vi "torreHanoi_v2.vi"() -> ()   [LabVIEW 2020]
uses:
  <vilib>/Analysis/Matrix/Datatypes/RealMatrix.ctl
  <vilib>/Utility/miscctls.llb/LVPositionTypeDef.ctl
  <vilib>/Utility/miscctls.llb/LVBoundsTypeDef.ctl
  <vilib>/Analysis/Matrix/NI_Matrix.lvlib
panel:
  out "PosAntPiezaCuatro":T1
  out "PosAntPiezaTres":T1
  out "PosAntPiezaDos":T1
  out "PosAntPiezaCinco":T1
  out "Posicion":i32
  out "Torre":i8
  out "posPiezaDos":i32[][](array[numeric])
  out "posPiezaTres":i32[][](array[numeric])
  out "posPiezaUno":i32[][](array[numeric])
  out "posPiezaCinco":i32[](array[numeric])
  out "posPiezaCuatro":i32[][](array[numeric])
  out "estadoTorreTres":i32[](array[numeric])
  out "estadoTorreUno":i32[](array[numeric])
  out "estadoTorreDos":i32[](array[numeric])
  out "PosAntPiezaUno":T1
  out "¿Pieza?":i8
  out "matrizPosIniciales":T2
  out "numMov":dbl
  out "minMov":dbl
  in  "numPiezas":enum16{"5", "4", "3"}(ring)
  in  "Iniciar":bool
  out "PiezaCinco":bool
  out "PiezaCuatro":bool
  out "PiezaTres":bool
  out "PiezaDos":bool
  in  "Deterner":bool
  out "PiezaUno":bool
  out "TorreUno":u8(slide) scale=0.0..100.0
  out "TorreDos":u8(slide) scale=0.0..100.0
  out "TorreTres":u8(slide) scale=0.0..100.0
  # "Número de Piezas"
  # "Minimo de Movimientos"
  # "Tus Movimientos"
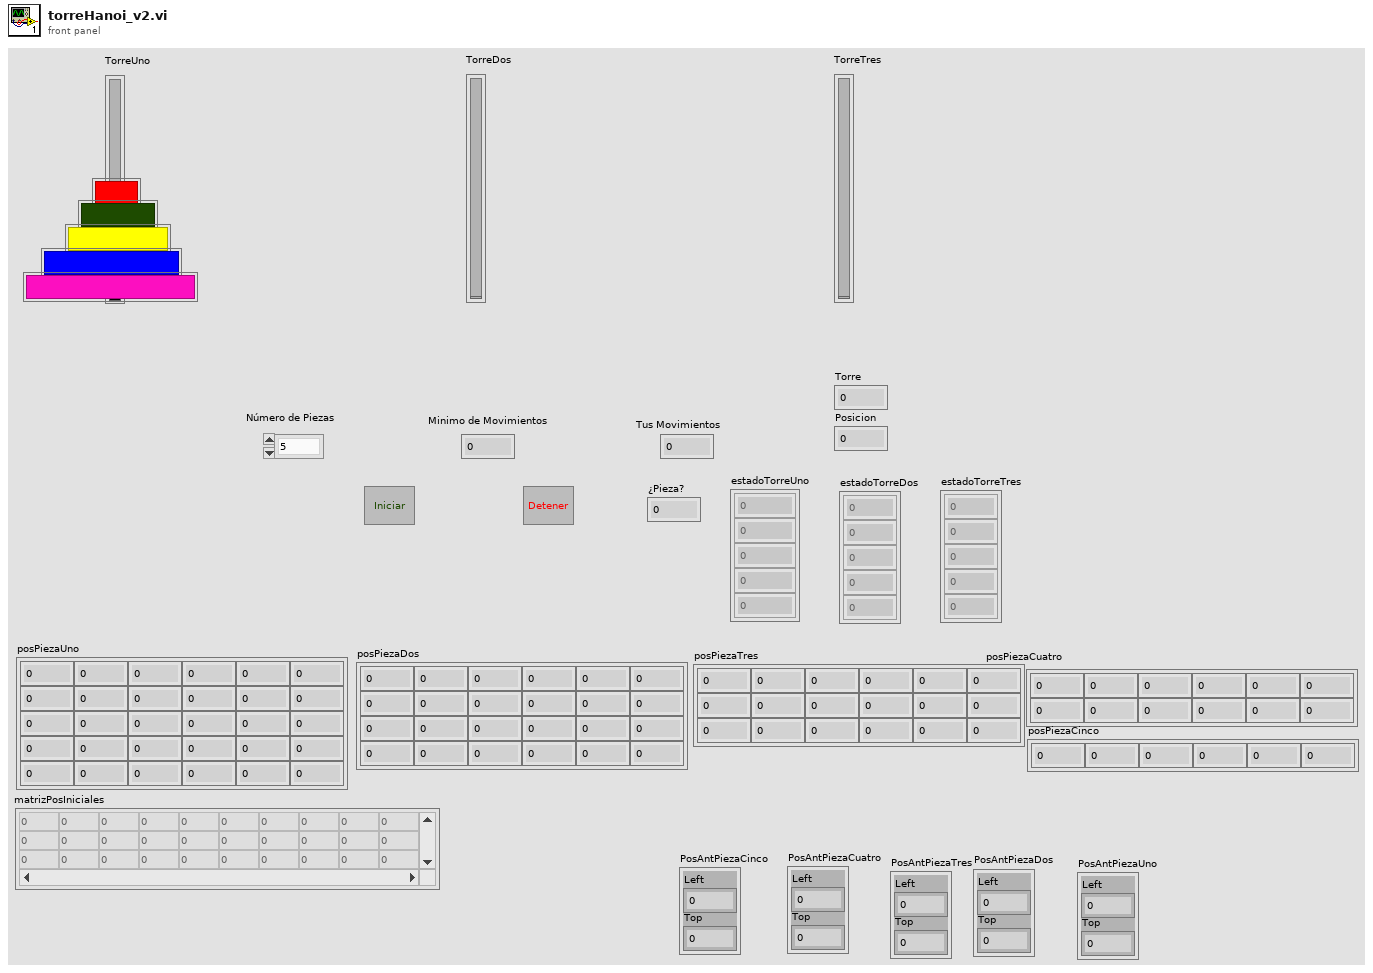
[diagram p1: front panel]
types:
  T1 = typedef "LVPositionTypeDef.ctl" = cluster{"Left":i32, "Top":i32}
  T2 = typedef "NI_Matrix.lvlib/RealMatrix.ctl" = dbl[][]
  T3 = typedef "LVBoundsTypeDef.ctl" = cluster{"Width":u32, "Height":u32}
  T4 = typedef "LVPoint32TypeDef.ctl" = cluster{"Horizontal":i32, "Vertical":i32}
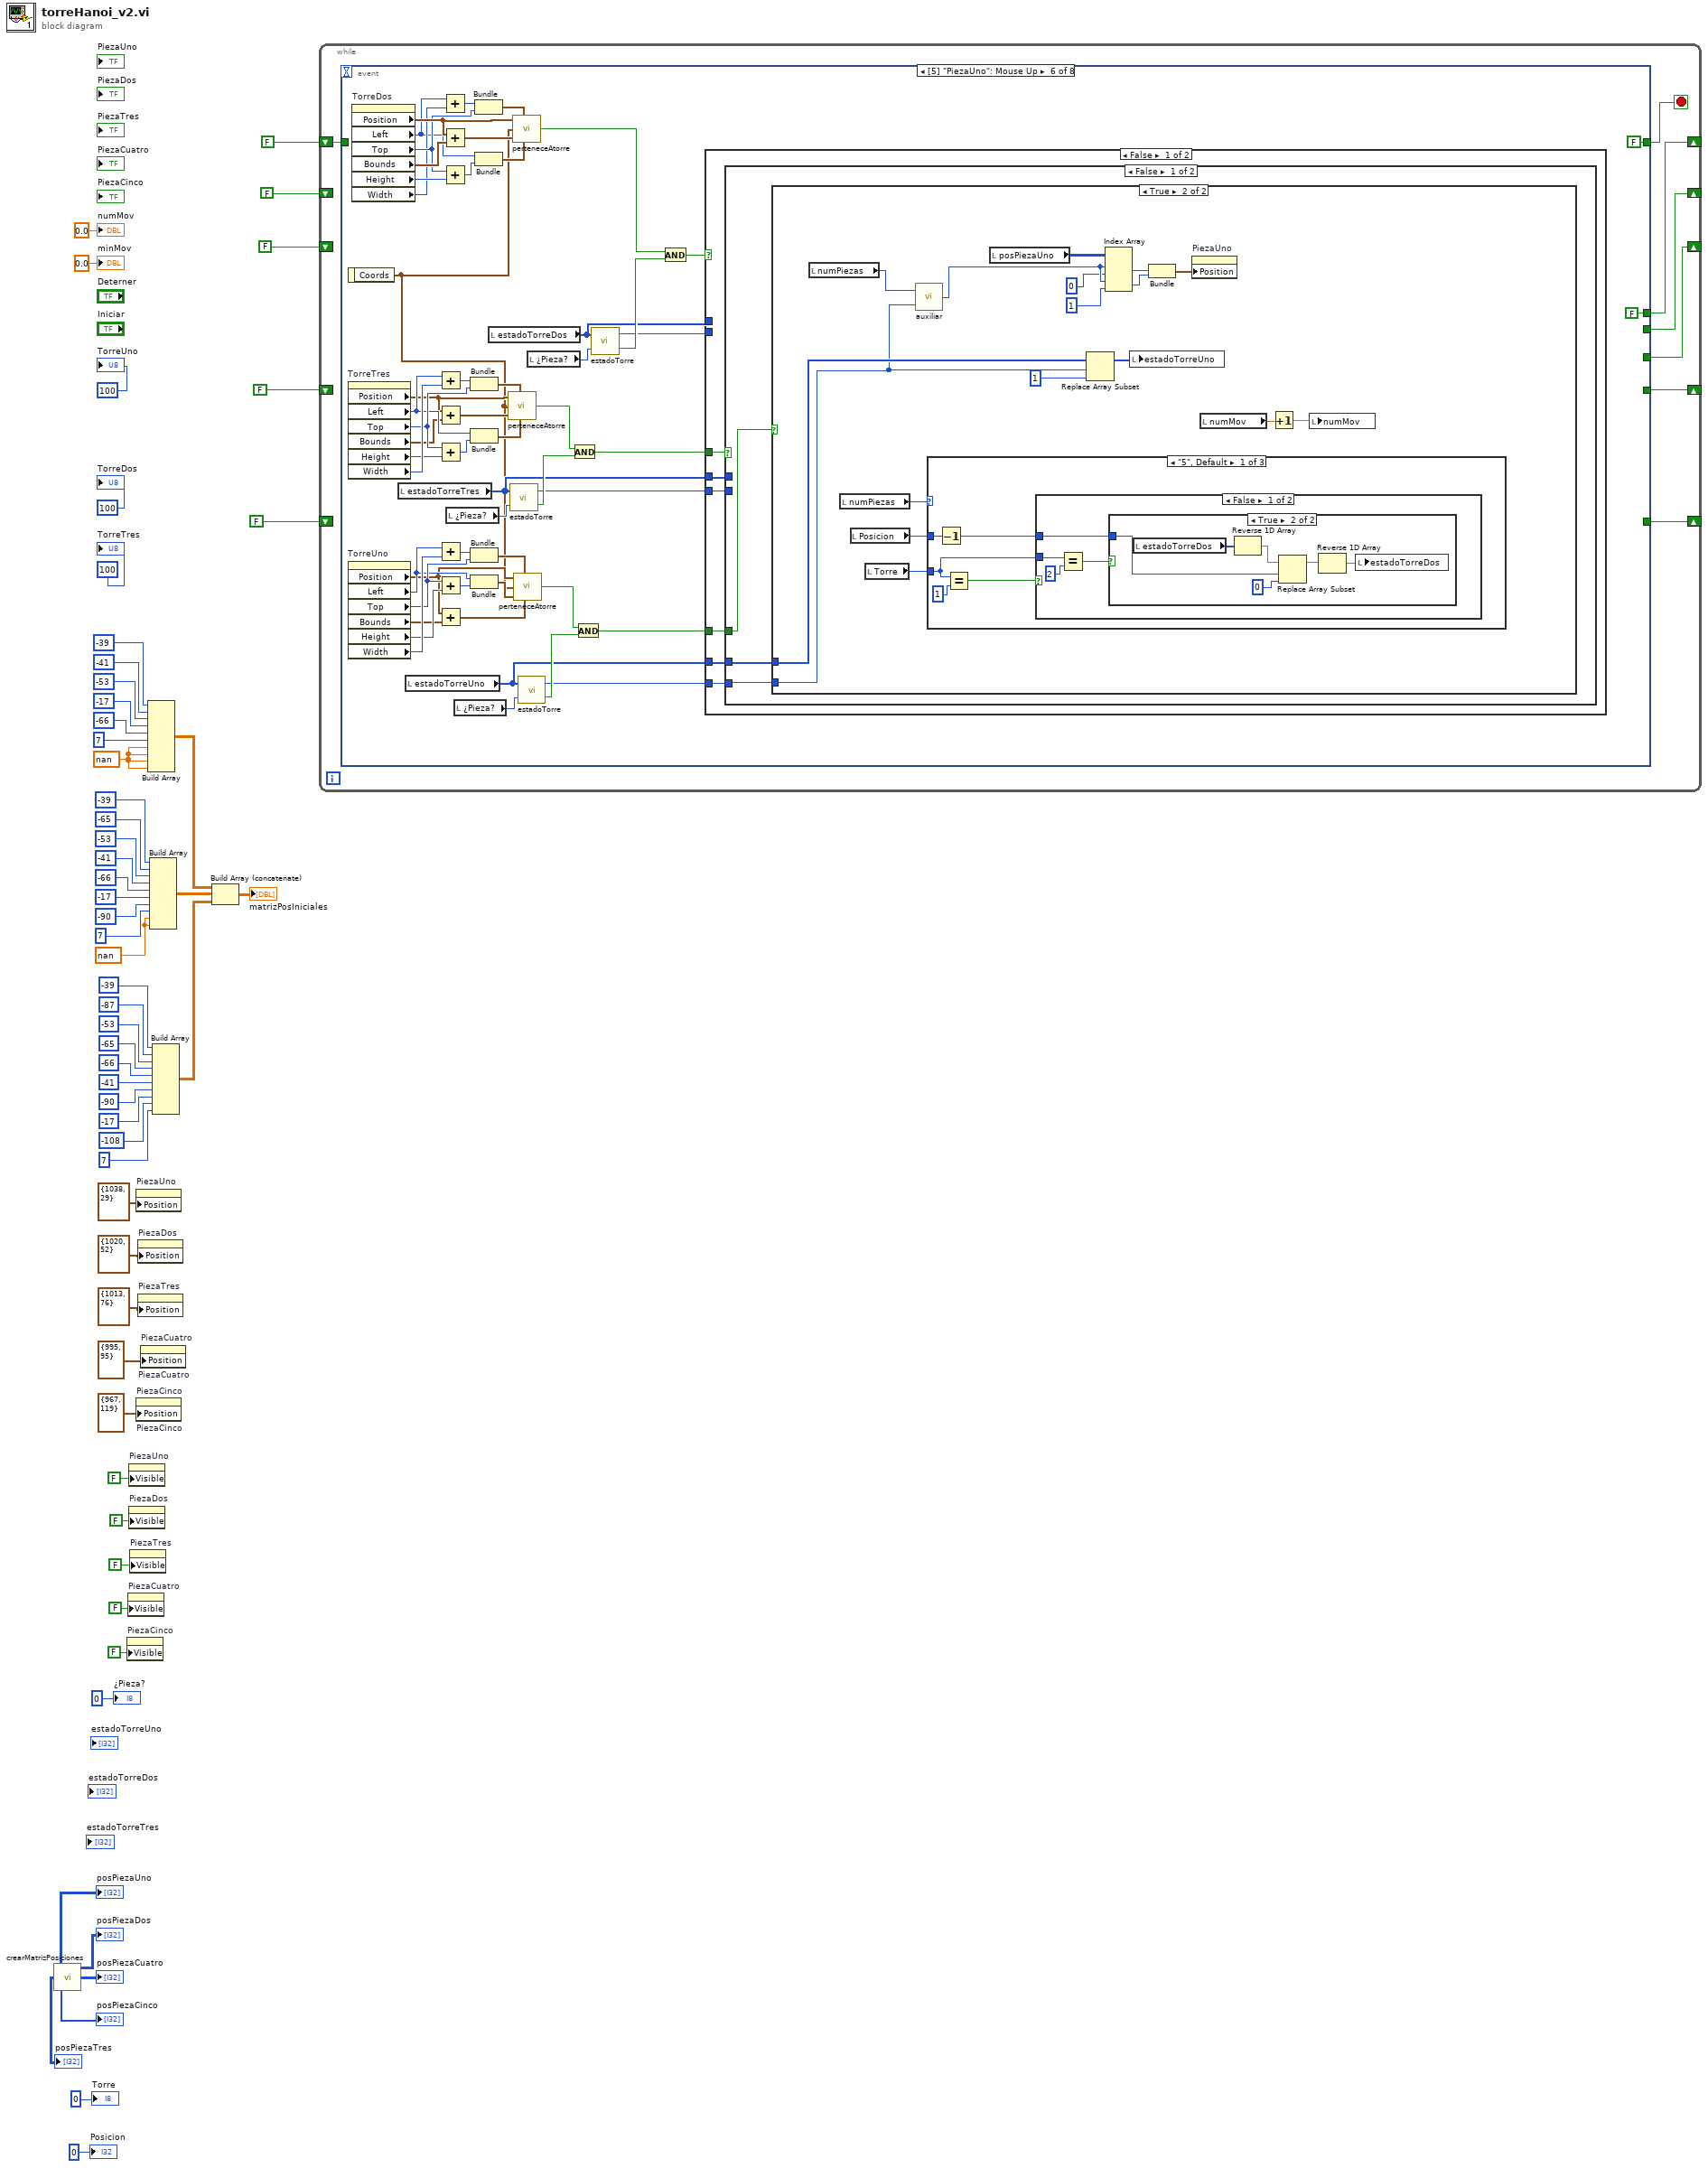
[diagram p0: block diagram]
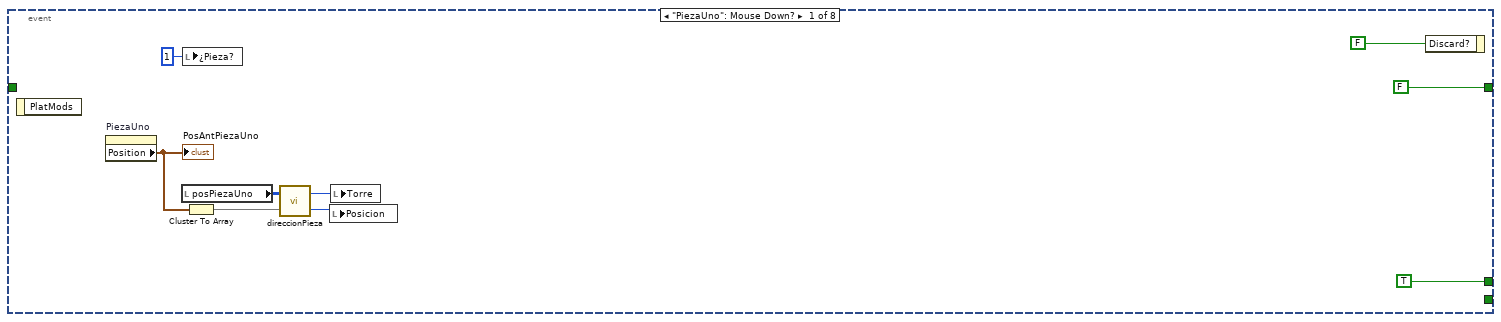
[diagram p2: hidden frame]
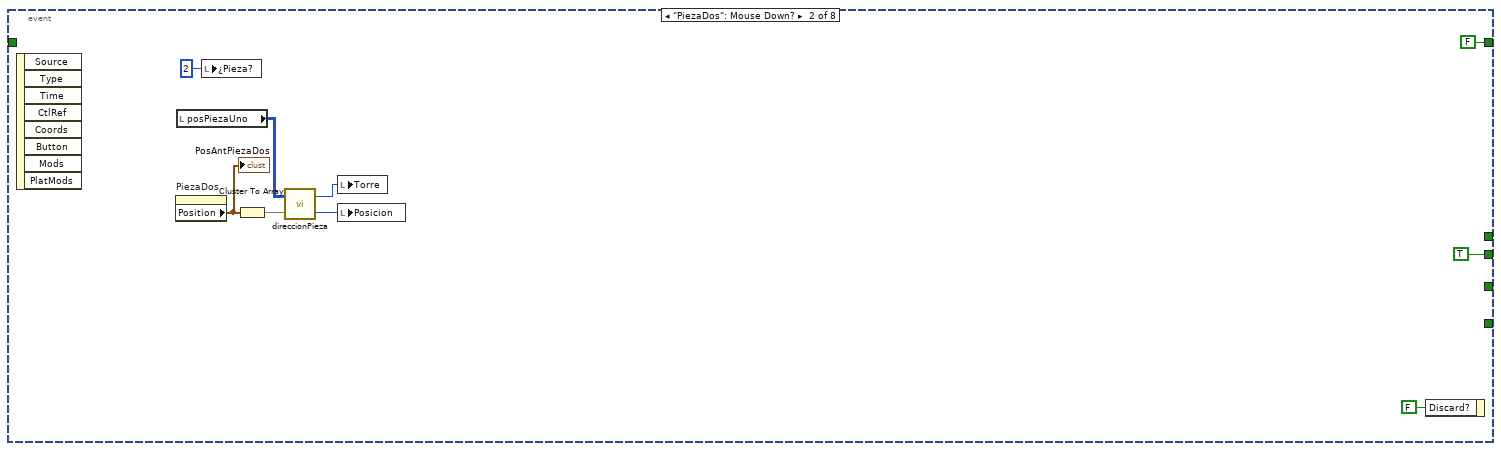
[diagram p3: hidden frame]
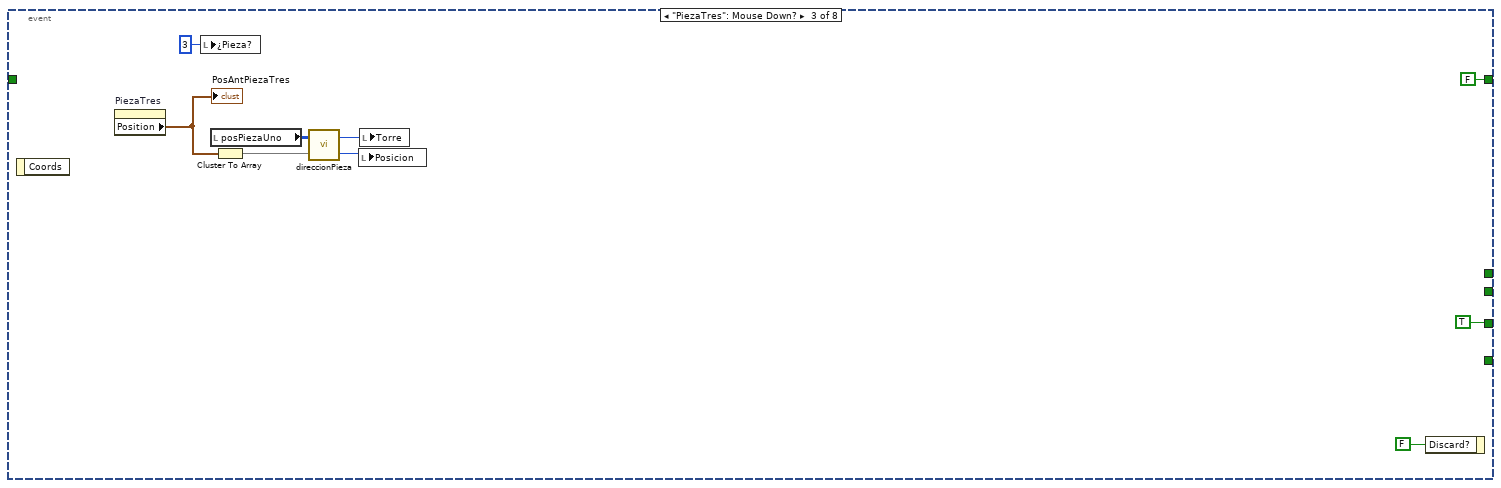
[diagram p4: hidden frame]
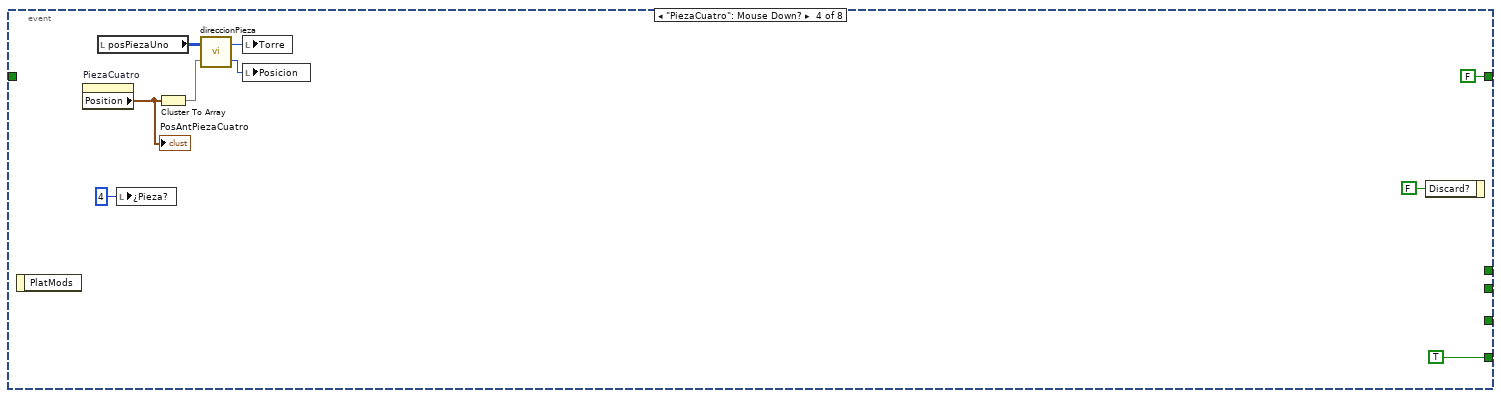
[diagram p5: hidden frame]
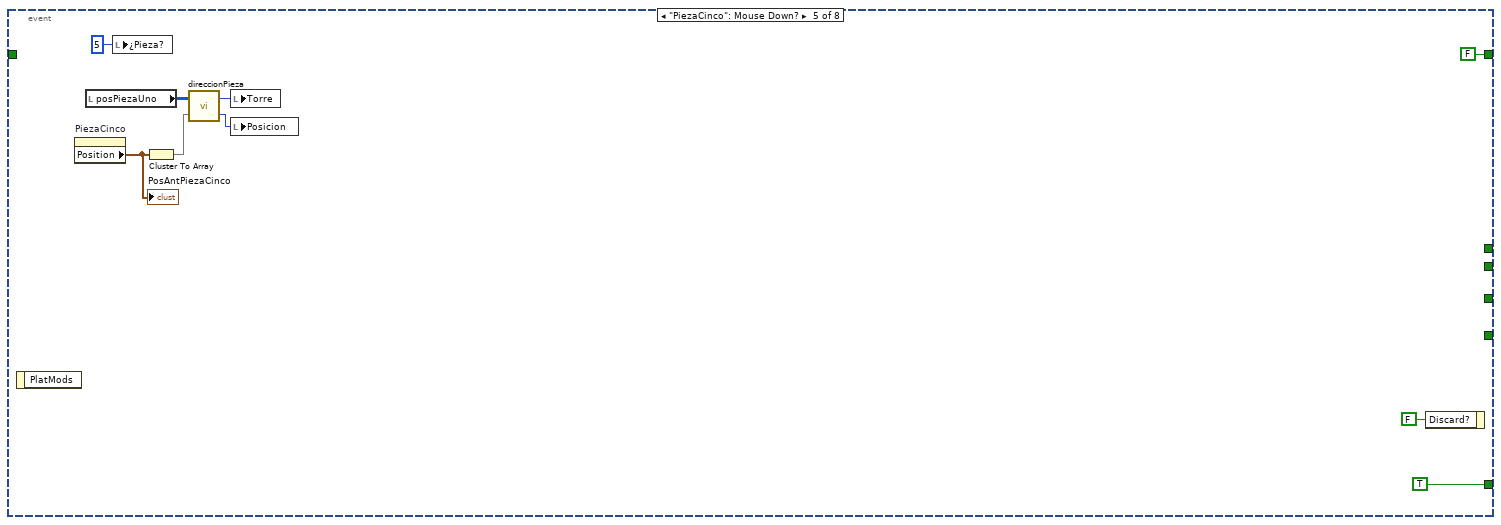
[diagram p6: hidden frame]
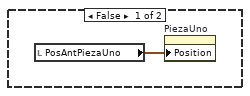
[diagram p7: hidden frame]
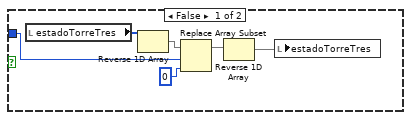
[diagram p8: hidden frame]
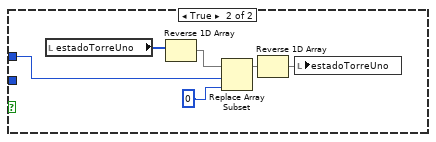
[diagram p9: hidden frame]
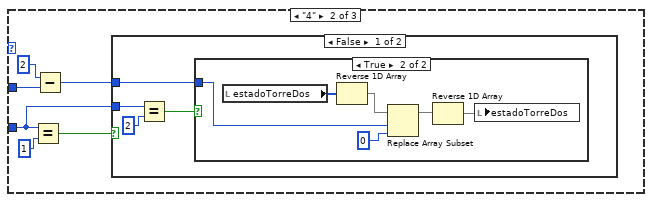
[diagram p10: hidden frame]
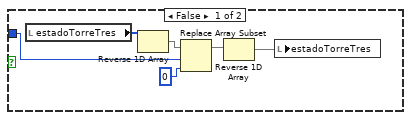
[diagram p11: hidden frame]
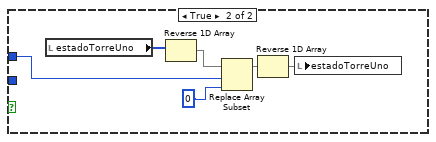
[diagram p12: hidden frame]
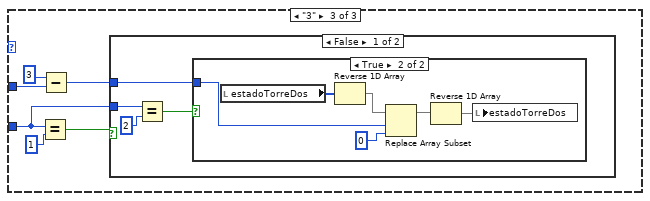
[diagram p13: hidden frame]
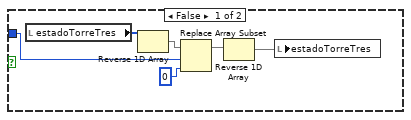
[diagram p14: hidden frame]
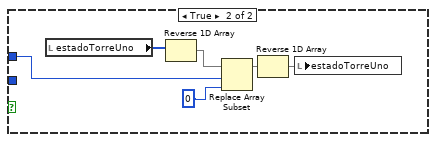
[diagram p15: hidden frame]
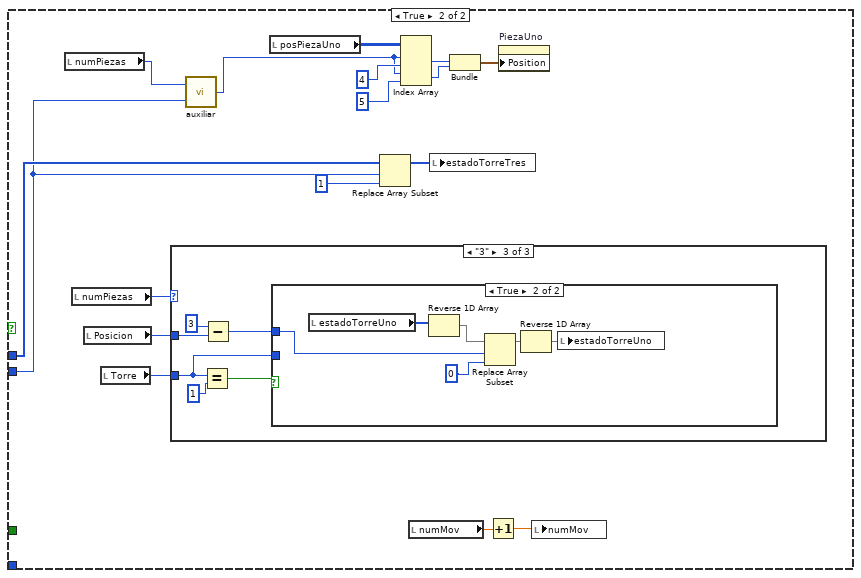
[diagram p16: hidden frame]
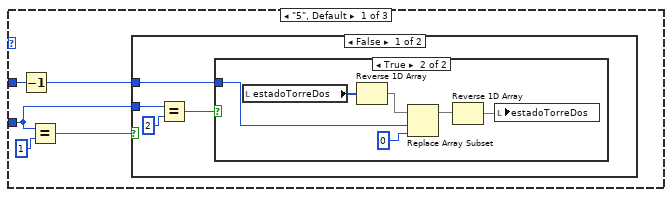
[diagram p17: hidden frame]
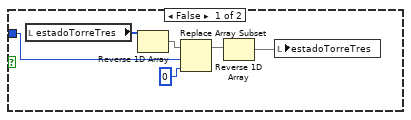
[diagram p18: hidden frame]
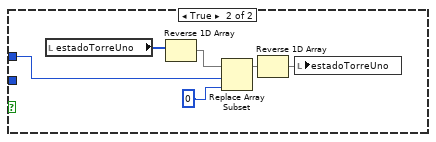
[diagram p19: hidden frame]
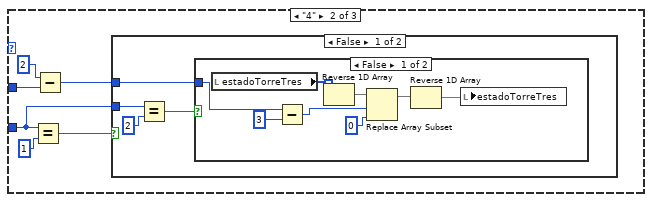
[diagram p20: hidden frame]
diagram:
  w41 = nan
  w50 = nan
  n1 = call "crearMatrizPosiciones.vi"() -> ("posPiezaCuatro"=→"posPiezaCuatro":i32[][], "posPiezaDos"=→"posPiezaDos":i32[][], "posPiezaCinco"=→"posPiezaCinco":i32[], "posPiezaTres"=→"posPiezaTres":i32[][], "posPiezaUno"=→"posPiezaUno":i32[][])  [unwired: 1 in]
  n2 = property on="PiezaCinco" class="Bool (strict)"("Visible"=FALSE ("PiezaCinco")) -> ()  [unwired: 2 in, 2 out]
  n3 = property on="PiezaCuatro" class="Bool (strict)"("Visible"=FALSE ("PiezaCuatro")) -> ()  [unwired: 2 in, 2 out]
  n4 = property on="PiezaUno" class="Bool (strict)"("Visible"=FALSE) -> ()  [unwired: 2 in, 2 out]
  n5 = property on="PiezaDos" class="Bool (strict)"("Visible"=FALSE ("PiezaDos")) -> ()  [unwired: 2 in, 2 out]
  n6 = property on="PiezaTres" class="Bool (strict)"("Visible"=FALSE) -> ()  [unwired: 2 in, 2 out]
  n7 = property on="PiezaUno" class="Bool (strict)"("Position"=T1 {"Left"=1038, "Top"=29}) -> ()  [unwired: 2 in, 2 out]
  n8 = property on="PiezaCinco" class="Bool (strict)"("Position"=T1 {"Left"=967, "Top"=119}) -> ()  [unwired: 2 in, 2 out]
  n9 = property on="PiezaCinco" class="Bool (strict)"("Position"=T1 {"Left"=967, "Top"=119}) -> ()  [unwired: 2 in, 2 out]
  n10 = property on="PiezaDos" class="Bool (strict)"("Position"=T1 {"Left"=1020, "Top"=52}) -> ()  [unwired: 2 in, 2 out]
  n11 = property on="PiezaTres" class="Bool (strict)"("Position"=T1 {"Left"=1013, "Top"=76}) -> ()  [unwired: 2 in, 2 out]
  n12 = property on="PiezaCuatro" class="Bool (strict)"("Position"=T1 {"Left"=995, "Top"=95}) -> ()  [unwired: 2 in, 2 out]
  n13 = property on="PiezaCuatro" class="Bool (strict)"("Position"=T1 {"Left"=995, "Top"=95}) -> ()  [unwired: 2 in, 2 out]
  n14 = Build Array(-39, -41 ("element"), -53 ("element"), -17 ("element"), -66 ("element"), 7 ("element"), w50, w50, w50, w50) -> (w30:T2)
  n15 = Build Array(-39, -65 ("element"), -53 ("element"), -41 ("element"), -66 ("element"), -17 ("element"), -90 ("element"), 7 ("element"), w41, w41) -> (w29:T2)
  n16 = Build Array(-39, -87 ("element"), -53 ("element"), -65 ("element"), -66 ("element"), -41 ("element"), -90 ("element"), -17 ("element"), -108 ("element"), 7 ("element")) -> (w28:T2)
  n17 = Build Array (concatenate)(w30, w29, w28) -> (→"matrizPosIniciales":T2)
  n18 = while {
    shift-right: [w66] -> _
    shift-left: FALSE -> [w65]
    shift-right: [w64] -> _
    shift-left: FALSE -> [_]
    shift-right: [w63] -> _
    shift-left: FALSE -> [_]
    shift-right: [w62] -> _
    shift-left: FALSE -> [_]
    shift-right: [w61] -> _
    shift-left: FALSE -> [_]
    stop <- w67 stop-if-true
    n19 = event shown="[5] \"PiezaUno\": Mouse Up" {
      selector: _ -> [_ _ _ _ _ _ _ _]
      dyn-events: _ -> [_ _ _ _ _ _ _ _]
      timeout: _ -> [_ _ _ _ _ _ _ _]
      tunnel: [FALSE FALSE FALSE FALSE FALSE FALSE FALSE _] -> w67
      tunnel: [TRUE _ _ _ _ FALSE w480 _] -> w66
      tunnel: w65 -> [_ _ _ _ _ _ w480 _]
      tunnel: [_ TRUE _ _ _ _ _ _] -> w64
      tunnel: [_ _ TRUE _ _ _ _ _] -> w63
      tunnel: [_ _ _ TRUE _ _ _ _] -> w62
      tunnel: [_ _ _ _ TRUE _ _ _] -> w61
      event "PiezaUno": Mouse Down? {
        n20 = event-data() -> ()  [unwired: 1 in, 1 out]
        n21 = property on="PiezaUno" class="Bool (strict)"() -> ("Position"=w72:T1)  [unwired: 2 in, 2 out]
        "PosAntPiezaUno" <- w72
        n22 = local read "posPiezaUno"() -> (w70:i32[][])
        n23 = local write "¿Pieza?"(i8 1 ("¿Pieza?")) -> ()
        n24 = Cluster To Array(cluster=w72) -> (array=w71:i32[])
        n25 = call "direccionPieza.vi"("posicion"=w71, "matrizPosiciones"=w70) -> ("Posicion"=w69:i32, "Torre"=w68:i8)
        n26 = local write "Posicion"(w69) -> ()
        n27 = local write "Torre"(w68) -> ()
        n28 = event-data("Discard?"=FALSE) -> ()  [unwired: 1 in, 1 out]
      }
      event "PiezaDos": Mouse Down? {
        n29 = event-data() -> ()  [unwired: 1 in, 8 out]
        n30 = property on="PiezaDos" class="Bool (strict)"() -> ("Position"=w80:T1)  [unwired: 2 in, 2 out]
        "PosAntPiezaDos" <- w80
        n31 = local read "posPiezaUno"() -> (w82:i32[][])
        n32 = local write "¿Pieza?"(i8 2 ("¿Pieza?")) -> ()
        n33 = Cluster To Array(cluster=w80) -> (array=w81:i32[])
        n34 = call "direccionPieza.vi"("posicion"=w81, "matrizPosiciones"=w82) -> ("Posicion"=w83:i32, "Torre"=w84:i8)
        n35 = local write "Torre"(w84) -> ()
        n36 = local write "Posicion"(w83) -> ()
        n37 = event-data("Discard?"=FALSE) -> ()  [unwired: 1 in, 1 out]
      }
      event "PiezaTres": Mouse Down? {
        n38 = event-data() -> ()  [unwired: 1 in, 1 out]
        n39 = property on="PiezaTres" class="Bool (strict)"() -> ("Position"=w89:T1)  [unwired: 2 in, 2 out]
        "PosAntPiezaTres" <- w89
        n40 = local write "¿Pieza?"(i8 3 ("¿Pieza?")) -> ()
        n41 = local read "posPiezaUno"() -> (w91:i32[][])
        n42 = Cluster To Array(cluster=w89) -> (array=w90:i32[])
        n43 = call "direccionPieza.vi"("posicion"=w90, "matrizPosiciones"=w91) -> ("Posicion"=w92:i32, "Torre"=w93:i8)
        n44 = local write "Posicion"(w92) -> ()
        n45 = local write "Torre"(w93) -> ()
        n46 = event-data("Discard?"=FALSE) -> ()  [unwired: 1 in, 1 out]
      }
      event "PiezaCuatro": Mouse Down? {
        n47 = event-data() -> ()  [unwired: 1 in, 1 out]
        n48 = property on="PiezaCuatro" class="Bool (strict)"() -> ("Position"=w99:T1)  [unwired: 2 in, 2 out]
        "PosAntPiezaCuatro" <- w99
        n49 = local read "posPiezaUno"() -> (w101:i32[][])
        n50 = local write "¿Pieza?"(i8 4 ("¿Pieza?")) -> ()
        n51 = Cluster To Array(cluster=w99) -> (array=w100:i32[])
        n52 = call "direccionPieza.vi"("posicion"=w100, "matrizPosiciones"=w101) -> ("Posicion"=w102:i32, "Torre"=w103:i8)
        n53 = local write "Torre"(w103) -> ()
        n54 = local write "Posicion"(w102) -> ()
        n55 = event-data("Discard?"=FALSE) -> ()  [unwired: 1 in, 1 out]
      }
      event "PiezaCinco": Mouse Down? {
        n56 = event-data() -> ()  [unwired: 1 in, 1 out]
        n57 = property on="PiezaCinco" class="Bool (strict)"() -> ("Position"=w107:T1)  [unwired: 2 in, 2 out]
        "PosAntPiezaCinco" <- w107
        n58 = local read "posPiezaUno"() -> (w110:i32[][])
        n59 = local write "¿Pieza?"(i8 5 ("¿Pieza?")) -> ()
        n60 = Cluster To Array(cluster=w107) -> (array=w109:i32[])
        n61 = call "direccionPieza.vi"("posicion"=w109, "matrizPosiciones"=w110) -> ("Posicion"=w111:i32, "Torre"=w112:i8)
        n62 = local write "Torre"(w112) -> ()
        n63 = local write "Posicion"(w111) -> ()
        n64 = event-data("Discard?"=FALSE) -> ()  [unwired: 1 in, 1 out]
      }
      event "PiezaUno": Mouse Up {
        n65 = event-data() -> ("Coords"=w119:T4)  [unwired: 1 in]
        n66 = property on="TorreTres" class="Slide (strict)"() -> ("Position"=w138:T1, "Left"=w141:i32, "Top"=w144:i32, "Bounds"=w139:T3, "Height"=w143:u32, "Width"=w147:u32)  [unwired: 2 in, 2 out]
        n67 = property on="TorreUno" class="Slide (strict)"() -> ("Position"=w122:T1, "Left"=w124:i32, "Top"=w127:i32, "Bounds"=w121:T3, "Height"=w126:u32, "Width"=w130:u32)  [unwired: 2 in, 2 out]
        n68 = property on="TorreDos" class="Slide (strict)"() -> ("Position"=w161:T1, "Left"=w156:i32, "Top"=w159:i32, "Bounds"=w162:T3, "Height"=w158:u32, "Width"=w157:u32)  [unwired: 2 in, 2 out]
        n69 = local read "estadoTorreTres"() -> (w132:i32[])
        n70 = local read "estadoTorreUno"() -> (w113:i32[])
        n71 = Add(x=w141, y=w147) -> (x+y=w146:u32)
        n72 = Add(x=w138, y=w139) -> (x+y=w137:T3)
        n73 = Add(x=w144, y=w143) -> (x+y=w142:u32)
        n74 = Add(x=w124, y=w130) -> (x+y=w128:u32)
        n75 = Add(x=w127, y=w126) -> (x+y=w125:u32)
        n76 = Add(x=w122, y=w121) -> (x+y=w120:T3)
        n77 = Add(x=w156, y=w157) -> (x+y=w164:u32)
        n78 = Add(x=w161, y=w162) -> (x+y=w160:T3)
        n79 = Add(x=w159, y=w158) -> (x+y=w155:u32)
        n80 = local read "¿Pieza?"() -> (w136:i8)
        n81 = local read "¿Pieza?"() -> (w118:i8)
        n82 = Bundle(w146, "Top"=w144) -> (w145:cluster{u32, "Top":i32})  [unwired: 1 in]
        n83 = Bundle("Left"=w141, w142) -> (w140:cluster{"Left":i32, u32})  [unwired: 1 in]
        n84 = Bundle(w128, "Top"=w127) -> (w129:cluster{u32, "Top":i32})  [unwired: 1 in]
        n85 = Bundle("Left"=w124, w125) -> (w123:cluster{"Left":i32, u32})  [unwired: 1 in]
        n86 = Bundle(w164, "Top"=w159) -> (w163:cluster{u32, "Top":i32})  [unwired: 1 in]
        n87 = Bundle("Left"=w156, w155) -> (w154:cluster{"Left":i32, u32})  [unwired: 1 in]
        n88 = local read "estadoTorreDos"() -> (w148:i32[])
        n89 = call "perteneceAtorre.vi"("P1"=w138, "P2"=w145, "P"=w119, "P3"=w137, "P4"=w140) -> ("out"=w135:bool)
        n90 = call "estadoTorre.vi"("¿pieza?"=w136, "estadoTorre"=w132) -> ("¿disponible?"=w134:bool, "posicionCero"=w133:i32)
        n91 = call "perteneceAtorre.vi"("P1"=w161, "P2"=w163, "P"=w119, "P3"=w160, "P4"=w154) -> ("out"=w152:bool)
        n92 = call "perteneceAtorre.vi"("P1"=w122, "P2"=w129, "P"=w119, "P3"=w123, "P4"=w120) -> ("out"=w117:bool)
        n93 = call "estadoTorre.vi"("¿pieza?"=w118, "estadoTorre"=w113) -> ("¿disponible?"=w116:bool, "posicionCero"=w114:i32)
        n94 = local read "¿Pieza?"() -> (w151:i8)
        n95 = And(x=w135, y=w134) -> (x .and. y?=w131:bool)
        n96 = And(x=w117, y=w116) -> (x .and. y?=w115:bool)
        n97 = call "estadoTorre.vi"("¿pieza?"=w151, "estadoTorre"=w148) -> ("¿disponible?"=w150:bool, "posicionCero"=w149:i32)
        n98 = And(x=w152, y=w150) -> (x .and. y?=w153:bool)
        n99 = case shown="False" w153 {
          tunnel: w149 -> [_ w385]
          tunnel: w148 -> [_ w389]
          tunnel: w133 -> [w170 _]
          tunnel: w132 -> [w171 _]
          tunnel: w131 -> [w172 _]
          tunnel: w115 -> [w169 _]
          tunnel: w114 -> [w167 _]
          tunnel: w113 -> [w168 _]
          frame False {
            n100 = case shown="False" w172 {
              tunnel: w171 -> [_ w283]
              tunnel: w170 -> [_ w282]
              tunnel: w169 -> [w175 _]
              tunnel: w168 -> [w174 _]
              tunnel: w167 -> [w173 _]
              frame False {
                n101 = case shown="True" w175 {
                  tunnel: w174 -> [_ w183]
                  tunnel: w173 -> [_ w182]
                  frame False {
                    n102 = local read "PosAntPiezaUno"() -> (w176:T1)
                    n103 = property on="PiezaUno" class="Bool (strict)"("Position"=w176) -> ()  [unwired: 2 in, 2 out]
                  }
                  frame True {
                    n104 = local read "numPiezas"() -> (w188:enum16{"5", "4", "3"})
                    n105 = local read "numPiezas"() -> (w181:enum16{"5", "4", "3"})
                    n106 = local read "Posicion"() -> (w180:i32)
                    n107 = local read "Torre"() -> (w179:i8)
                    n108 = call "auxiliar.vi"("posicion"=w182, "numPiezas"=w188) -> ("posicion"=w187:i32)
                    n109 = case shown="\"5\", Default" w181 {
                      tunnel: w180 -> [w198 w224 w252]
                      tunnel: w179 -> [w195 w221 w249]
                      frame "5", Default {
                        n110 = Decrement(x=w198) -> (x-1=w194:i32)
                        n111 = Equal?(x=w195, y=i8 1) -> (x = y?=w196:bool)
                        n112 = case shown="False" w196 {
                          tunnel: w194 -> [w199 w219]
                          tunnel: w195 -> [w202 _]
                          frame False {
                            n113 = Equal?(x=w202, y=i8 2) -> (x = y?=w200:bool)
                            n114 = case shown="True" w200 {
                              tunnel: w199 -> [w207 w213]
                              frame False {
                                n115 = local read "estadoTorreTres"() -> (w204:i32[])
                                n116 = Reverse 1D Array(array=w204) -> (reversed array=w203:i32[])
                                n117 = Replace Array Subset(array=w203, new element=0 ("new element/subarray"), index=w207) -> (w206:i32[])
                                n118 = Reverse 1D Array(array=w206) -> (reversed array=w205:i32[])
                                n119 = local write "estadoTorreTres"(w205) -> ()
                              }
                              frame True {
                                n120 = local read "estadoTorreDos"() -> (w210:i32[])
                                n121 = Reverse 1D Array(array=w210) -> (reversed array=w209:i32[])
                                n122 = Replace Array Subset(array=w209, new element=0 ("new element/subarray"), index=w213) -> (w212:i32[])
                                n123 = Reverse 1D Array(array=w212) -> (reversed array=w211:i32[])
                                n124 = local write "estadoTorreDos"(w211) -> ()
                              }
                            }
                          }
                          frame True {
                            n125 = local read "estadoTorreUno"() -> (w216:i32[])
                            n126 = Reverse 1D Array(array=w216) -> (reversed array=w215:i32[])
                            n127 = Replace Array Subset(array=w215, new element=0 ("new element/subarray"), index=w219) -> (w218:i32[])
                            n128 = Reverse 1D Array(array=w218) -> (reversed array=w217:i32[])
                            n129 = local write "estadoTorreUno"(w217) -> ()
                          }
                        }
                      }
                      frame "4" {
                        n130 = Equal?(x=w221, y=i8 1) -> (x = y?=w226:bool)
                        n131 = Subtract(x=2, y=w224) -> (x-y=w223:i32)
                        n132 = case shown="False" w226 {
                          tunnel: w223 -> [w228 w247]
                          tunnel: w221 -> [w227 _]
                          frame False {
                            n133 = Equal?(x=w227, y=i8 2) -> (x = y?=w229:bool)
                            n134 = case shown="True" w229 {
                              tunnel: w228 -> [w235 w241]
                              frame False {
                                n135 = local read "estadoTorreTres"() -> (w232:i32[])
                                n136 = Reverse 1D Array(array=w232) -> (reversed array=w231:i32[])
                                n137 = Replace Array Subset(array=w231, new element=0 ("new element/subarray"), index=w235) -> (w234:i32[])
                                n138 = Reverse 1D Array(array=w234) -> (reversed array=w233:i32[])
                                n139 = local write "estadoTorreTres"(w233) -> ()
                              }
                              frame True {
                                n140 = local read "estadoTorreDos"() -> (w238:i32[])
                                n141 = Reverse 1D Array(array=w238) -> (reversed array=w237:i32[])
                                n142 = Replace Array Subset(array=w237, new element=0 ("new element/subarray"), index=w241) -> (w240:i32[])
                                n143 = Reverse 1D Array(array=w240) -> (reversed array=w239:i32[])
                                n144 = local write "estadoTorreDos"(w239) -> ()
                              }
                            }
                          }
                          frame True {
                            n145 = local read "estadoTorreUno"() -> (w244:i32[])
                            n146 = Reverse 1D Array(array=w244) -> (reversed array=w243:i32[])
                            n147 = Replace Array Subset(array=w243, new element=0 ("new element/subarray"), index=w247) -> (w246:i32[])
                            n148 = Reverse 1D Array(array=w246) -> (reversed array=w245:i32[])
                            n149 = local write "estadoTorreUno"(w245) -> ()
                          }
                        }
                      }
                      frame "3" {
                        n150 = Equal?(x=w249, y=i8 1) -> (x = y?=w254:bool)
                        n151 = Subtract(x=3, y=w252) -> (x-y=w250:i32)
                        n152 = case shown="False" w254 {
                          tunnel: w250 -> [w256 w275]
                          tunnel: w249 -> [w255 _]
                          frame False {
                            n153 = Equal?(x=w255, y=i8 2) -> (x = y?=w257:bool)
                            n154 = case shown="True" w257 {
                              tunnel: w256 -> [w263 w269]
                              frame False {
                                n155 = local read "estadoTorreTres"() -> (w260:i32[])
                                n156 = Reverse 1D Array(array=w260) -> (reversed array=w259:i32[])
                                n157 = Replace Array Subset(array=w259, new element=0 ("new element/subarray"), index=w263) -> (w262:i32[])
                                n158 = Reverse 1D Array(array=w262) -> (reversed array=w261:i32[])
                                n159 = local write "estadoTorreTres"(w261) -> ()
                              }
                              frame True {
                                n160 = local read "estadoTorreDos"() -> (w266:i32[])
                                n161 = Reverse 1D Array(array=w266) -> (reversed array=w265:i32[])
                                n162 = Replace Array Subset(array=w265, new element=0 ("new element/subarray"), index=w269) -> (w268:i32[])
                                n163 = Reverse 1D Array(array=w268) -> (reversed array=w267:i32[])
                                n164 = local write "estadoTorreDos"(w267) -> ()
                              }
                            }
                          }
                          frame True {
                            n165 = local read "estadoTorreUno"() -> (w272:i32[])
                            n166 = Reverse 1D Array(array=w272) -> (reversed array=w271:i32[])
                            n167 = Replace Array Subset(array=w271, new element=0 ("new element/subarray"), index=w275) -> (w274:i32[])
                            n168 = Reverse 1D Array(array=w274) -> (reversed array=w273:i32[])
                            n169 = local write "estadoTorreUno"(w273) -> ()
                          }
                        }
                      }
                    }
                    n170 = local read "posPiezaUno"() -> (w192:i32[][])
                    n171 = Replace Array Subset(array=w183, new element=1, index=w182) -> (w193:i32[])
                    n172 = Index Array(array=w192, index (row) #1=w187, index (col) #1=0 ("disabled index (col)"), index (row) #2=w187, index (col) #2=1 ("disabled index (col)")) -> (element #1=w191:i32, element #2=w189:i32)
                    n173 = local write "estadoTorreUno"(w193) -> ()
                    n174 = Bundle(w191, w189) -> (w190:cluster{i32, i32})  [unwired: 1 in]
                    n175 = property on="PiezaUno" class="Bool (strict)"("Position"=w190) -> ()  [unwired: 2 in, 2 out]
                    n176 = local read "numMov"() -> (w178:dbl)
                    n177 = Increment(x=w178) -> (x+1=w177:dbl)
                    n178 = local write "numMov"(w177) -> ()
                  }
                }
              }
              frame True {
                n179 = local read "numPiezas"() -> (w285:enum16{"5", "4", "3"})
                n180 = local read "numPiezas"() -> (w281:enum16{"5", "4", "3"})
                n181 = local read "Posicion"() -> (w280:i32)
                n182 = local read "Torre"() -> (w279:i8)
                n183 = case shown="\"3\"" w281 {
                  tunnel: w280 -> [w298 w324 w354]
                  tunnel: w279 -> [w295 w321 w351]
                  frame "5", Default {
                    n184 = Decrement(x=w298) -> (x-1=w294:i32)
                    n185 = Equal?(x=w295, y=i8 1) -> (x = y?=w296:bool)
                    n186 = case shown="False" w296 {
                      tunnel: w294 -> [w299 w319]
                      tunnel: w295 -> [w302 _]
                      frame False {
                        n187 = Equal?(x=w302, y=i8 2) -> (x = y?=w300:bool)
                        n188 = case shown="True" w300 {
                          tunnel: w299 -> [w307 w313]
                          frame False {
                            n189 = local read "estadoTorreTres"() -> (w304:i32[])
                            n190 = Reverse 1D Array(array=w304) -> (reversed array=w303:i32[])
                            n191 = Replace Array Subset(array=w303, new element=0 ("new element/subarray"), index=w307) -> (w306:i32[])
                            n192 = Reverse 1D Array(array=w306) -> (reversed array=w305:i32[])
                            n193 = local write "estadoTorreTres"(w305) -> ()
                          }
                          frame True {
                            n194 = local read "estadoTorreDos"() -> (w310:i32[])
                            n195 = Reverse 1D Array(array=w310) -> (reversed array=w309:i32[])
                            n196 = Replace Array Subset(array=w309, new element=0 ("new element/subarray"), index=w313) -> (w312:i32[])
                            n197 = Reverse 1D Array(array=w312) -> (reversed array=w311:i32[])
                            n198 = local write "estadoTorreDos"(w311) -> ()
                          }
                        }
                      }
                      frame True {
                        n199 = local read "estadoTorreUno"() -> (w316:i32[])
                        n200 = Reverse 1D Array(array=w316) -> (reversed array=w315:i32[])
                        n201 = Replace Array Subset(array=w315, new element=0 ("new element/subarray"), index=w319) -> (w318:i32[])
                        n202 = Reverse 1D Array(array=w318) -> (reversed array=w317:i32[])
                        n203 = local write "estadoTorreUno"(w317) -> ()
                      }
                    }
                  }
                  frame "4" {
                    n204 = Equal?(x=w321, y=i8 1) -> (x = y?=w326:bool)
                    n205 = Subtract(x=2, y=w324) -> (x-y=w323:i32)
                    n206 = case shown="False" w326 {
                      tunnel: w323 -> [w328 w349]
                      tunnel: w321 -> [w327 _]
                      frame False {
                        n207 = Equal?(x=w327, y=i8 2) -> (x = y?=w329:bool)
                        n208 = case shown="False" w329 {
                          tunnel: w328 -> [w337 w343]
                          frame False {
                            n209 = local read "estadoTorreTres"() -> (w332:i32[])
                            n210 = Subtract(x=w337, y=3) -> (x-y=w335:i32)
                            n211 = Reverse 1D Array(array=w332) -> (reversed array=w331:i32[])
                            n212 = Replace Array Subset(array=w331, new element=0 ("new element/subarray"), index=w335) -> (w334:i32[])
                            n213 = Reverse 1D Array(array=w334) -> (reversed array=w333:i32[])
                            n214 = local write "estadoTorreTres"(w333) -> ()
                          }
                          frame True {
                            n215 = local read "estadoTorreDos"() -> (w340:i32[])
                            n216 = Reverse 1D Array(array=w340) -> (reversed array=w339:i32[])
                            n217 = Replace Array Subset(array=w339, new element=0 ("new element/subarray"), index=w343) -> (w342:i32[])
                            n218 = Reverse 1D Array(array=w342) -> (reversed array=w341:i32[])
                            n219 = local write "estadoTorreDos"(w341) -> ()
                          }
                        }
                      }
                      frame True {
                        n220 = local read "estadoTorreUno"() -> (w346:i32[])
                        n221 = Reverse 1D Array(array=w346) -> (reversed array=w345:i32[])
                        n222 = Replace Array Subset(array=w345, new element=0 ("new element/subarray"), index=w349) -> (w348:i32[])
                        n223 = Reverse 1D Array(array=w348) -> (reversed array=w347:i32[])
                        n224 = local write "estadoTorreUno"(w347) -> ()
                      }
                    }
                  }
                  frame "3" {
                    n225 = Equal?(x=w351, y=i8 1) -> (x = y?=w356:bool)
                    n226 = Subtract(x=3, y=w354) -> (x-y=w352:i32)
                    n227 = case shown="True" w356 {
                      tunnel: w352 -> [w358 w377]
                      tunnel: w351 -> [w357 _]
                      frame False {
                        n228 = Equal?(x=w357, y=i8 2) -> (x = y?=w359:bool)
                        n229 = case shown="False" w359 {
                          tunnel: w358 -> [w365 w371]
                          frame False {
                            n230 = local read "estadoTorreTres"() -> (w362:i32[])
                            n231 = Reverse 1D Array(array=w362) -> (reversed array=w361:i32[])
                            n232 = Replace Array Subset(array=w361, new element=0 ("new element/subarray"), index=w365) -> (w364:i32[])
                            n233 = Reverse 1D Array(array=w364) -> (reversed array=w363:i32[])
                            n234 = local write "estadoTorreTres"(w363) -> ()
                          }
                          frame True {
                            n235 = local read "estadoTorreDos"() -> (w368:i32[])
                            n236 = Reverse 1D Array(array=w368) -> (reversed array=w367:i32[])
                            n237 = Replace Array Subset(array=w367, new element=0 ("new element/subarray"), index=w371) -> (w370:i32[])
                            n238 = Reverse 1D Array(array=w370) -> (reversed array=w369:i32[])
                            n239 = local write "estadoTorreDos"(w369) -> ()
                          }
                        }
                      }
                      frame True {
                        n240 = local read "estadoTorreUno"() -> (w374:i32[])
                        n241 = Reverse 1D Array(array=w374) -> (reversed array=w373:i32[])
                        n242 = Replace Array Subset(array=w373, new element=0 ("new element/subarray"), index=w377) -> (w376:i32[])
                        n243 = Reverse 1D Array(array=w376) -> (reversed array=w375:i32[])
                        n244 = local write "estadoTorreUno"(w375) -> ()
                      }
                    }
                  }
                }
                n245 = call "auxiliar.vi"("posicion"=w282, "numPiezas"=w285) -> ("posicion"=w284:i32)
                n246 = local read "posPiezaUno"() -> (w291:i32[][])
                n247 = Replace Array Subset(array=w283, new element=1, index=w282) -> (w292:i32[])
                n248 = Index Array(array=w291, index (row) #1=w284, index (col) #1=4 ("disabled index (col)"), index (row) #2=w284, index (col) #2=5 ("disabled index (col)")) -> (element #1=w288:i32, element #2=w286:i32)
                n249 = local read "numMov"() -> (w278:dbl)
                n250 = local write "estadoTorreTres"(w292) -> ()
                n251 = Bundle(w288, w286) -> (w287:cluster{i32, i32})  [unwired: 1 in]
                n252 = Increment(x=w278) -> (x+1=w277:dbl)
                n253 = property on="PiezaUno" class="Bool (strict)"("Position"=w287) -> ()  [unwired: 2 in, 2 out]
                n254 = local write "numMov"(w277) -> ()
              }
            }
          }
          frame True {
            n255 = local read "numPiezas"() -> (w383:enum16{"5", "4", "3"})
            n256 = local read "numPiezas"() -> (w386:enum16{"5", "4", "3"})
            n257 = local read "Posicion"() -> (w382:i32)
            n258 = local read "Torre"() -> (w381:i8)
            n259 = case shown="\"4\"" w383 {
              tunnel: w382 -> [w400 w426 w454]
              tunnel: w381 -> [w397 w423 w451]
              frame "5", Default {
                n260 = Decrement(x=w400) -> (x-1=w396:i32)
                n261 = Equal?(x=w397, y=i8 1) -> (x = y?=w398:bool)
                n262 = case shown="False" w398 {
                  tunnel: w396 -> [w401 w421]
                  tunnel: w397 -> [w404 _]
                  frame False {
                    n263 = Equal?(x=w404, y=i8 2) -> (x = y?=w402:bool)
                    n264 = case shown="True" w402 {
                      tunnel: w401 -> [w409 w415]
                      frame False {
                        n265 = local read "estadoTorreTres"() -> (w406:i32[])
                        n266 = Reverse 1D Array(array=w406) -> (reversed array=w405:i32[])
                        n267 = Replace Array Subset(array=w405, new element=0 ("new element/subarray"), index=w409) -> (w408:i32[])
                        n268 = Reverse 1D Array(array=w408) -> (reversed array=w407:i32[])
                        n269 = local write "estadoTorreTres"(w407) -> ()
                      }
                      frame True {
                        n270 = local read "estadoTorreDos"() -> (w412:i32[])
                        n271 = Reverse 1D Array(array=w412) -> (reversed array=w411:i32[])
                        n272 = Replace Array Subset(array=w411, new element=0 ("new element/subarray"), index=w415) -> (w414:i32[])
                        n273 = Reverse 1D Array(array=w414) -> (reversed array=w413:i32[])
                        n274 = local write "estadoTorreDos"(w413) -> ()
                      }
                    }
                  }
                  frame True {
                    n275 = local read "estadoTorreUno"() -> (w418:i32[])
                    n276 = Reverse 1D Array(array=w418) -> (reversed array=w417:i32[])
                    n277 = Replace Array Subset(array=w417, new element=0 ("new element/subarray"), index=w421) -> (w420:i32[])
                    n278 = Reverse 1D Array(array=w420) -> (reversed array=w419:i32[])
                    n279 = local write "estadoTorreUno"(w419) -> ()
                  }
                }
              }
              frame "4" {
                n280 = Equal?(x=w423, y=i8 1) -> (x = y?=w428:bool)
                n281 = Subtract(x=2, y=w426) -> (x-y=w425:i32)
                n282 = case shown="False" w428 {
                  tunnel: w425 -> [w430 w449]
                  tunnel: w423 -> [w429 _]
                  frame False {
                    n283 = Equal?(x=w429, y=i8 2) -> (x = y?=w431:bool)
                    n284 = case shown="True" w431 {
                      tunnel: w430 -> [w437 w443]
                      frame False {
                        n285 = local read "estadoTorreTres"() -> (w434:i32[])
                        n286 = Reverse 1D Array(array=w434) -> (reversed array=w433:i32[])
                        n287 = Replace Array Subset(array=w433, new element=0 ("new element/subarray"), index=w437) -> (w436:i32[])
                        n288 = Reverse 1D Array(array=w436) -> (reversed array=w435:i32[])
                        n289 = local write "estadoTorreTres"(w435) -> ()
                      }
                      frame True {
                        n290 = local read "estadoTorreDos"() -> (w440:i32[])
                        n291 = Reverse 1D Array(array=w440) -> (reversed array=w439:i32[])
                        n292 = Replace Array Subset(array=w439, new element=0 ("new element/subarray"), index=w443) -> (w442:i32[])
                        n293 = Reverse 1D Array(array=w442) -> (reversed array=w441:i32[])
                        n294 = local write "estadoTorreDos"(w441) -> ()
                      }
                    }
                  }
                  frame True {
                    n295 = local read "estadoTorreUno"() -> (w446:i32[])
                    n296 = Reverse 1D Array(array=w446) -> (reversed array=w445:i32[])
                    n297 = Replace Array Subset(array=w445, new element=0 ("new element/subarray"), index=w449) -> (w448:i32[])
                    n298 = Reverse 1D Array(array=w448) -> (reversed array=w447:i32[])
                    n299 = local write "estadoTorreUno"(w447) -> ()
                  }
                }
              }
              frame "3" {
                n300 = Equal?(x=w451, y=i8 1) -> (x = y?=w456:bool)
                n301 = Subtract(x=3, y=w454) -> (x-y=w452:i32)
                n302 = case shown="False" w456 {
                  tunnel: w452 -> [w458 w477]
                  tunnel: w451 -> [w457 _]
                  frame False {
                    n303 = Equal?(x=w457, y=i8 2) -> (x = y?=w459:bool)
                    n304 = case shown="True" w459 {
                      tunnel: w458 -> [w465 w471]
                      frame False {
                        n305 = local read "estadoTorreTres"() -> (w462:i32[])
                        n306 = Reverse 1D Array(array=w462) -> (reversed array=w461:i32[])
                        n307 = Replace Array Subset(array=w461, new element=0 ("new element/subarray"), index=w465) -> (w464:i32[])
                        n308 = Reverse 1D Array(array=w464) -> (reversed array=w463:i32[])
                        n309 = local write "estadoTorreTres"(w463) -> ()
                      }
                      frame True {
                        n310 = local read "estadoTorreDos"() -> (w468:i32[])
                        n311 = Reverse 1D Array(array=w468) -> (reversed array=w467:i32[])
                        n312 = Replace Array Subset(array=w467, new element=0 ("new element/subarray"), index=w471) -> (w470:i32[])
                        n313 = Reverse 1D Array(array=w470) -> (reversed array=w469:i32[])
                        n314 = local write "estadoTorreDos"(w469) -> ()
                      }
                    }
                  }
                  frame True {
                    n315 = local read "estadoTorreUno"() -> (w474:i32[])
                    n316 = Reverse 1D Array(array=w474) -> (reversed array=w473:i32[])
                    n317 = Replace Array Subset(array=w473, new element=0 ("new element/subarray"), index=w477) -> (w476:i32[])
                    n318 = Reverse 1D Array(array=w476) -> (reversed array=w475:i32[])
                    n319 = local write "estadoTorreUno"(w475) -> ()
                  }
                }
              }
            }
            n320 = call "auxiliar.vi"("posicion"=w385, "numPiezas"=w386) -> ("posicion"=w384:i32)
            n321 = local read "posPiezaUno"() -> (w393:i32[][])
            n322 = Replace Array Subset(array=w389, new element=1, index=w385) -> (w394:i32[])
            n323 = Index Array(array=w393, index (row) #1=w384, index (col) #1=2 ("disabled index (col)"), index (row) #2=w384, index (col) #2=3 ("disabled index (col)")) -> (element #1=w390:i32, element #2=w387:i32)
            n324 = local write "estadoTorreDos"(w394) -> ()
            n325 = local read "numMov"() -> (w380:dbl)
            n326 = Bundle(w390, w387) -> (w388:cluster{i32, i32})  [unwired: 1 in]
            n327 = property on="PiezaUno" class="Bool (strict)"("Position"=w388) -> ()  [unwired: 2 in, 2 out]
            n328 = Increment(x=w380) -> (x+1=w379:dbl)
            n329 = local write "numMov"(w379) -> ()
          }
        }
      }
      event Mouse Move {
        n330 = event-data() -> ("Coords"=w481:T4)  [unwired: 1 in]
        n331 = case shown="True" w480 {
          tunnel: w481 -> [_ w483]
          frame False {
          }
          frame True {
            n332 = property on="PiezaUno" class="Bool (strict)"() -> ("Bounds"=w486:T3)  [unwired: 2 in, 2 out]
            n333 = Divide(x=w486, y=T3 {"Width"=2, "Height"=2}) -> (x/y=w484:cluster{"Width":dbl, "Height":dbl})
            n334 = Subtract(x=w483, y=w484) -> (x-y=w482:cluster{dbl, dbl})
            n335 = property on="PiezaUno" class="Bool (strict)"("Position"=w482) -> ()  [unwired: 2 in, 2 out]
          }
        }
      }
      event "Iniciar": Value Change {
        n336 = event-data() -> ()  [unwired: 1 in, 6 out]
        n337 = case shown="\"5\"" "numPiezas" {
          frame "3", Default {
            w515 = 0 ("index (row)")
            n338 = local read "matrizPosIniciales"() -> (w518:T2)
            n339 = local write "minMov"(7.0 ("minMov")) -> ()
            n340 = Index Array(array=w518, index (row) #1=w515, index (col) #1=w515, index (row) #2=w515, index (col) #2=1 ("disabled index (col)"), index (row) #3=w515, index (col) #3=2 ("disabled index (col)"), index (row) #4=w515, index (col) #4=3 ("disabled index (col)"), index (row) #5=w515, index (col) #5=4 ("disabled index (col)"), index (row) #6=w515, index (col) #6=5 ("disabled index (col)")) -> (element #1=w511:dbl, element #2=w510:dbl, element #3=w509:dbl, element #4=w508:dbl, element #5=w507:dbl, element #6=w506:dbl)
            n341 = property on="PiezaUno" class="Bool (strict)"("Left"=w511, "Top"=w510) -> ()  [unwired: 2 in, 2 out]
            n342 = property on="PiezaDos" class="Bool (strict)"("Left"=w509, "Top"=w508) -> ()  [unwired: 2 in, 2 out]
            n343 = property on="PiezaTres" class="Bool (strict)"("Left"=w507, "Top"=w506) -> ()  [unwired: 2 in, 2 out]
            n344 = Initialize Array(0, 3 ("dimension size")) -> (w496:i32[])
            n345 = local write "estadoTorreDos"(w496) -> ()
            n346 = local write "estadoTorreTres"(w496) -> ()
            n347 = Replace Array Subset(array=w496, new element #1=3 ("new element/subarray"), index #1=0 ("index"), new element #2=2 ("new element/subarray"), index #2=1 ("index"), new element #3=1 ("new element/subarray"), index #3=2 ("index")) -> (w489:i32[])
            n348 = local write "estadoTorreUno"(w489) -> ()
            n349 = property on="PiezaCinco" class="Bool (strict)"("Visible"=FALSE ("PiezaCinco")) -> ()  [unwired: 2 in, 2 out]
            n350 = property on="PiezaCuatro" class="Bool (strict)"("Visible"=FALSE ("PiezaCuatro")) -> ()  [unwired: 2 in, 2 out]
            n351 = property on="PiezaUno" class="Bool (strict)"("Visible"=TRUE) -> ()  [unwired: 2 in, 2 out]
            n352 = property on="PiezaDos" class="Bool (strict)"("Visible"=TRUE ("PiezaDos")) -> ()  [unwired: 2 in, 2 out]
            n353 = property on="PiezaTres" class="Bool (strict)"("Visible"=TRUE) -> ()  [unwired: 2 in, 2 out]
            n354 = property on="PiezaCinco" class="Bool (strict)"("Position"=T1 {"Left"=967, "Top"=119}) -> ()  [unwired: 2 in, 2 out]
            n355 = property on="PiezaCuatro" class="Bool (strict)"("Position"=T1 {"Left"=995, "Top"=95}) -> ()  [unwired: 2 in, 2 out]
          }
          frame "4" {
            w552 = 1
            n356 = local read "matrizPosIniciales"() -> (w554:T2)
            n357 = Initialize Array(0, 4 ("dimension size")) -> (w529:i32[])
            n358 = local write "estadoTorreDos"(w529) -> ()
            n359 = local write "estadoTorreTres"(w529) -> ()
            n360 = Replace Array Subset(array=w529, new element #1=4 ("new element/subarray"), index #1=0 ("index"), new element #2=3 ("new element/subarray"), index #2=1 ("index"), new element #3=2 ("new element/subarray"), index #3=2 ("index"), new element #4=1 ("new element/subarray"), index #4=3 ("index")) -> (w522:i32[])
            n361 = Index Array(array=w554, index (row) #1=w552, index (col) #1=0, index (row) #2=w552, index (col) #2=w552, index (row) #3=w552, index (col) #3=2, index (row) #4=w552, index (col) #4=3, index (row) #5=w552, index (col) #5=4, index (row) #6=w552, index (col) #6=5, index (row) #7=w552, index (col) #7=6, index (row) #8=w552, index (col) #8=7) -> (element #1=w545:dbl, element #2=w544:dbl, element #3=w543:dbl, element #4=w542:dbl, element #5=w541:dbl, element #6=w540:dbl, element #7=w539:dbl, element #8=w538:dbl)
            n362 = local write "estadoTorreUno"(w522) -> ()
            n363 = property on="PiezaUno" class="Bool (strict)"("Left"=w545, "Top"=w544) -> ()  [unwired: 2 in, 2 out]
            n364 = property on="PiezaDos" class="Bool (strict)"("Left"=w543, "Top"=w542) -> ()  [unwired: 2 in, 2 out]
            n365 = property on="PiezaTres" class="Bool (strict)"("Left"=w541, "Top"=w540) -> ()  [unwired: 2 in, 2 out]
            n366 = property on="PiezaCuatro" class="Bool (strict)"("Left"=w539, "Top"=w538) -> ()  [unwired: 2 in, 2 out]
            n367 = local write "minMov"(15.0 ("minMov")) -> ()
            n368 = property on="PiezaUno" class="Bool (strict)"("Visible"=TRUE) -> ()  [unwired: 2 in, 2 out]
            n369 = property on="PiezaCinco" class="Bool (strict)"("Visible"=FALSE ("PiezaCinco")) -> ()  [unwired: 2 in, 2 out]
            n370 = property on="PiezaCuatro" class="Bool (strict)"("Visible"=TRUE ("PiezaCuatro")) -> ()  [unwired: 2 in, 2 out]
            n371 = property on="PiezaDos" class="Bool (strict)"("Visible"=TRUE ("PiezaDos")) -> ()  [unwired: 2 in, 2 out]
            n372 = property on="PiezaTres" class="Bool (strict)"("Visible"=TRUE) -> ()  [unwired: 2 in, 2 out]
            n373 = property on="PiezaCinco" class="Bool (strict)"("Position"=T1 {"Left"=967, "Top"=119}) -> ()  [unwired: 2 in, 2 out]
          }
          frame "5" {
            w582 = 2
            n374 = local read "matrizPosIniciales"() -> (w595:T2)
            n375 = local write "minMov"(31.0 ("minMov")) -> ()
            n376 = Index Array(array=w595, index (row) #1=w582, index (col) #1=0, index (row) #2=w582, index (col) #2=1, index (row) #3=w582, index (col) #3=w582, index (row) #4=w582, index (col) #4=3, index (row) #5=w582, index (col) #5=4, index (row) #6=w582, index (col) #6=5, index (row) #7=w582, index (col) #7=6, index (row) #8=w582, index (col) #8=7, index (row) #9=w582, index (col) #9=8, index (row) #10=w582, index (col) #10=9) -> (element #1=w585:dbl, element #2=w584:dbl, element #3=w583:dbl, element #4=w581:dbl, element #5=w580:dbl, element #6=w579:dbl, element #7=w578:dbl, element #8=w577:dbl, element #9=w576:dbl, element #10=w575:dbl)
            n377 = property on="PiezaCinco" class="Bool (strict)"("Left"=w576, "Top"=w575) -> ()  [unwired: 2 in, 2 out]
            n378 = property on="PiezaUno" class="Bool (strict)"("Left"=w585, "Top"=w584) -> ()  [unwired: 2 in, 2 out]
            n379 = property on="PiezaTres" class="Bool (strict)"("Left"=w580, "Top"=w579) -> ()  [unwired: 2 in, 2 out]
            n380 = property on="PiezaCuatro" class="Bool (strict)"("Left"=w578, "Top"=w577) -> ()  [unwired: 2 in, 2 out]
            n381 = property on="PiezaDos" class="Bool (strict)"("Left"=w583, "Top"=w581) -> ()  [unwired: 2 in, 2 out]
            n382 = Initialize Array(0, 5 ("dimension size")) -> (w569:i32[])
            n383 = local write "estadoTorreDos"(w569) -> ()
            n384 = local write "estadoTorreTres"(w569) -> ()
            n385 = property on="PiezaCinco" class="Bool (strict)"("Visible"=TRUE ("PiezaCinco")) -> ()  [unwired: 2 in, 2 out]
            n386 = property on="PiezaCuatro" class="Bool (strict)"("Visible"=TRUE ("PiezaCuatro")) -> ()  [unwired: 2 in, 2 out]
            n387 = property on="PiezaDos" class="Bool (strict)"("Visible"=TRUE ("PiezaDos")) -> ()  [unwired: 2 in, 2 out]
            n388 = property on="PiezaTres" class="Bool (strict)"("Visible"=TRUE) -> ()  [unwired: 2 in, 2 out]
            n389 = property on="PiezaUno" class="Bool (strict)"("Visible"=TRUE) -> ()  [unwired: 2 in, 2 out]
            n390 = Replace Array Subset(array=w569, new element #1=5 ("new element/subarray"), index #1=0 ("index"), new element #2=4 ("new element/subarray"), index #2=1 ("index"), new element #3=3 ("new element/subarray"), index #3=2 ("index"), new element #4=2 ("new element/subarray"), index #4=3 ("new element/subarray"), new element #5=1 ("new element/subarray"), index #5=4 ("new element/subarray")) -> (w568:i32[])
            n391 = local write "estadoTorreUno"(w568) -> ()
          }
        }
      }
    }
  }
  "TorreUno" <- u8 100 ("TorreUno")
  "TorreDos" <- u8 100 ("TorreDos")
  "TorreTres" <- u8 100 ("TorreTres")
  "minMov" <- 0.0 ("minMov")
  "numMov" <- 0.0 ("numMov")
  "¿Pieza?" <- i8 0 ("¿Pieza?")
  "Torre" <- i8 0 ("Torre")
  "Posicion" <- 0 ("Posicion")
